vi "getLVProjBuildItems.vi"(8 "error in (no error)":errorcluster, 11 "Project Path":path caption="selected path") -> (0 "error out":errorcluster, 1 "Target Names":string[](array[string]), 2 "BuildSpec Names":string[][](array[string]), 3 "Project Path":path, 4 "BuildSpec Type":string[][](array[string]), 5 "Project Name":string)   [LabVIEW 2017, in "BuildServer.lvlib" / "BuildServer.lvclass"]
uses:
  BuildServer.lvclass
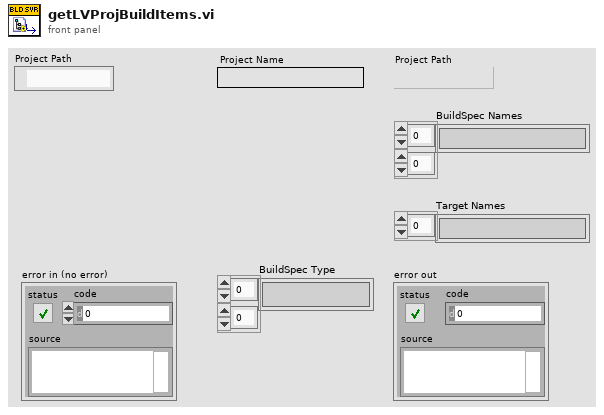
[diagram p1: front panel]
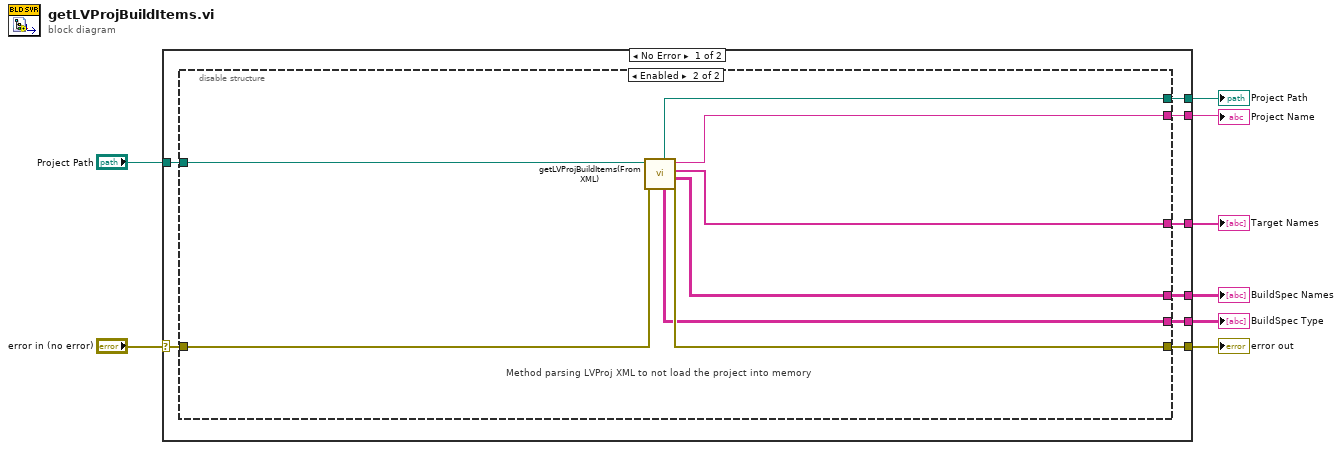
[diagram p0: block diagram]
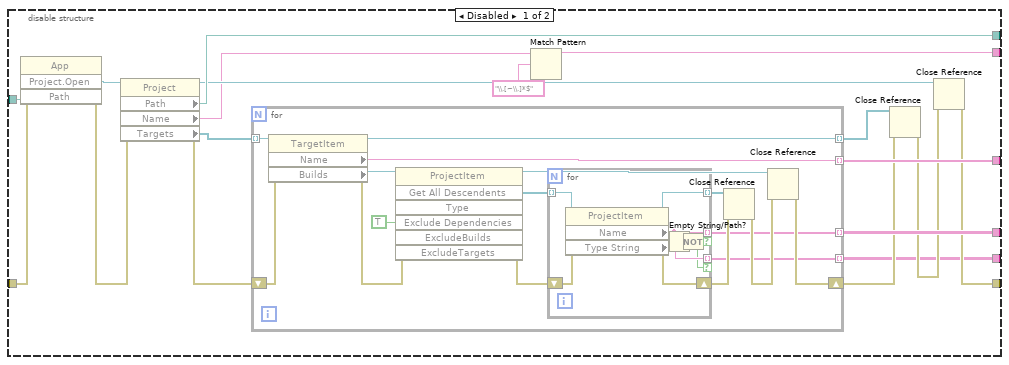
[diagram p2: hidden frame]
diagram:
  n1 = case shown="No Error" "error in (no error)" {
    selector: "error in (no error)" -> [w13 w67]
    tunnel: [w16 _] -> w8
    tunnel: [w15 _] -> w7
    tunnel: [w14 _] -> w6
    tunnel: "Project Path" -> [w12 _]
    tunnel: [w11 w67] -> w5
    tunnel: [w10 _] -> w4
    tunnel: [w9 _] -> w3
    frame No Error {
      n2 = disable-structure shown="Enabled" {
        disable-tunnel: [w34 w59] -> w16
        disable-tunnel: [w33 w60] -> w15
        disable-tunnel: [w32 w62] -> w14
        disable-tunnel: w13 -> [w31 w65]
        disable-tunnel: w12 -> [w28 w66]
        disable-tunnel: [w27 w64] -> w11
        disable-tunnel: [w20 w63] -> w10
        disable-tunnel: [w17 w61] -> w9
        frame Disabled {
          n3 = invoke class="App" method="Project.Open"(error in=w31, "Path"=w28) -> (error out=w30:errorcluster, "Project:Open"=w29:refnum<vi>)  [unwired: 2 in, 2 out]
          n4 = property class="Project"(reference=w29, error in=w30) -> (reference out=w24:refnum<vi>, error out=w22:errorcluster, "Path"=w32:path, "Name"=w19:string, "Targets"=w21:refnum<vi>[])
          n5 = for {
            tunnel: w21 -> [w50] mode=indexing
            tunnel: [w37] -> w34 mode=indexing
            shift-right: [w38] -> w26
            shift-left: w22 -> [w46]
            tunnel: [w43] -> w23 mode=indexing
            tunnel: [w36] -> w33 mode=indexing
            tunnel: [w35] -> w20 mode=indexing
            n6 = property class="TargetItem"(reference=w50, error in=w46) -> (reference out=w43:refnum<vi>, error out=w45:errorcluster, "Name"=w36:string, "Builds"=w49:refnum<vi>)
            n7 = invoke class="ProjectItem" method="Get All Descendents"(reference=w49, error in=w45, "Exclude Dependencies"=TRUE ("ExcludeDependencies")) -> (reference out=w41:refnum<vi>, error out=w44:errorcluster, "All Descendents"=w47:refnum<vi>[])  [unwired: 4 in, 4 out]
            n8 = for {
              tunnel: w47 -> [w58] mode=indexing
              tunnel: [w53] -> w37 mode=indexing if=w51
              shift-right: [w57] -> w39
              shift-left: w44 -> [w56]
              tunnel: [w55] -> w42 mode=indexing
              tunnel: [w52] -> w35 mode=indexing if=w51
              n9 = property class="ProjectItem"(reference=w58, error in=w56) -> (reference out=w55:refnum<vi>, error out=w57:errorcluster, "Name"=w53:string, "Type String"=w52:string)
              n10 = Empty String/Path?(string/path=w53) -> (empty?=w54:bool)
              n11 = Not(x=w54) -> (.not. x?=w51:bool)
            }
            n12 = Close Reference(reference=w42, error in (no error)=w39) -> (error out=w40:errorcluster)
            n13 = Close Reference(reference=w41, error in (no error)=w40) -> (error out=w38:errorcluster)
          }
          n14 = Match Pattern(string=w19, regular expression="\\.[~\\.]*$") -> (before substring=w17:string)  [unwired: 4 out]
          n15 = Close Reference(reference=w23, error in (no error)=w26) -> (error out=w25:errorcluster)
          n16 = Close Reference(reference=w24, error in (no error)=w25) -> (error out=w27:errorcluster)
        }
        frame Enabled {
          # "Method parsing LVProj XML to not load the project into memory"
          n17 = call "getLVProjBuildItems(From XML).vi"("error in (no error)"=w65, "Path"=w66) -> ("error out"=w64:errorcluster, "BuildSpec Names"=w59:string[][], "Target Names"=w60:string[], "Project Name"=w61:string, "BuildSpec Types"=w63:string[][], "Project Path"=w62:path)  [unwired: 4 in]
        }
      }
    }
    frame Error {
    }
  }
  "BuildSpec Names" <- w8
  "Target Names" <- w7
  "Project Name" <- w3
  "Project Path" <- w6
  "error out" <- w5
  "BuildSpec Type" <- w4
